vi "Agilent DMM Set Blank Screen.vi"(8 "error in (no error)":errorcluster, 10 "Blank Screen":bool, 11 "VISA Resource Name":refnum<visa-resource-name>) -> (0 "error out":errorcluster, 3 "dup VISA Resource Name":refnum<visa-resource-name>)   [LabVIEW 2011]
doc: "This VI for the HP 8753 is used to read the sweep type.\n\n0 LINEAR FREQ\n1 LOG FREQ\n2 LIST FREQ\n3 CW TIME\n4 POWER SWEEP"
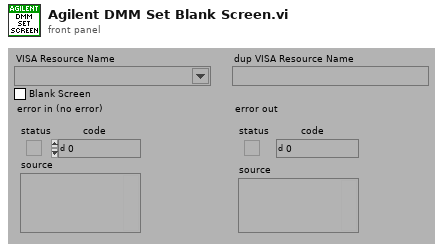
[diagram p1: front panel]
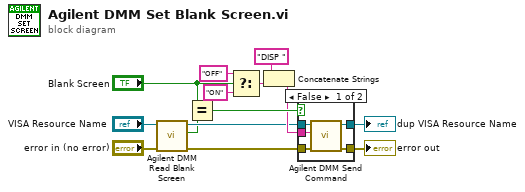
[diagram p0: block diagram]
diagram:
  n1 = call "Agilent DMM Read Blank Screen.vi"("error in (no error)"="error in (no error)", "VISA Resource Name"="VISA Resource Name") -> ("error out"=w4:errorcluster, "Blank Screen"=w1:bool, "dup VISA Resource Name"=w3:refnum<visa-resource-name>)  [unwired: 7 out]
  n2 = Equal?(x="Blank Screen", y=w1) -> (x = y?=w10:bool)
  n3 = Select(t="OFF" ("write buffer"), s="Blank Screen", f="ON" ("write buffer")) -> (s? t:f=w11:string)
  n4 = Concatenate Strings("DISP " ("string"), w11) -> (w7:string)
  n5 = case shown="False" w10 {
    tunnel: [w19 w21] -> w9
    tunnel: [w18 w20] -> w8
    tunnel: w7 -> [w17 _]
    tunnel: w3 -> [w16 w21]
    tunnel: w4 -> [w15 w20]
    frame False {
      n6 = call "Agilent DMM Send Command.vi"("error in (no error)"=w15, "Command"=w17, "VISA Resource Name"=w16) -> ("error out"=w18:errorcluster, "dup VISA Resource Name"=w19:refnum<visa-resource-name>)  [unwired: 2 in, 5 out]
    }
    frame True {
    }
  }
  "dup VISA Resource Name" <- w9
  "error out" <- w8
